vi "ModulationNiveaus.vi"() -> ()   [LabVIEW 2011]
panel:
  in  "max":dbl
  in  "min":dbl
  in  "harmonics":dbl
  in  "ModulationNiveaus":dbl[](array[numeric])
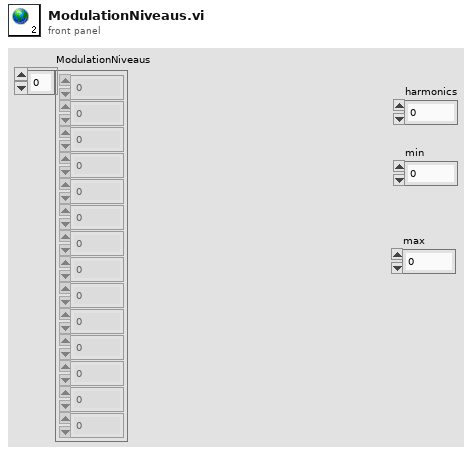
[diagram p1: front panel]
diagram:
